vi "SetFrameRate.vi"(8 "error in (no error)":errorcluster, 10 "Frame Rate":u8, 11 "CameraTestingBL in":refnum<class "CameraTesting.lvclass">) -> (0 "error out":errorcluster, 3 "CameraTestingBL out":refnum<class "CameraTesting.lvclass">)   [LabVIEW 2020, in "CameraTesting.lvlib" / "CameraTesting.lvclass"]
doc: "Set the frame rate of the camera"
uses:
  CameraTesting.lvclass
  CameraTesting.lvclass/CameraTesting.ctl
  Camera/ICamera/ICamera/ICamera.lvclass
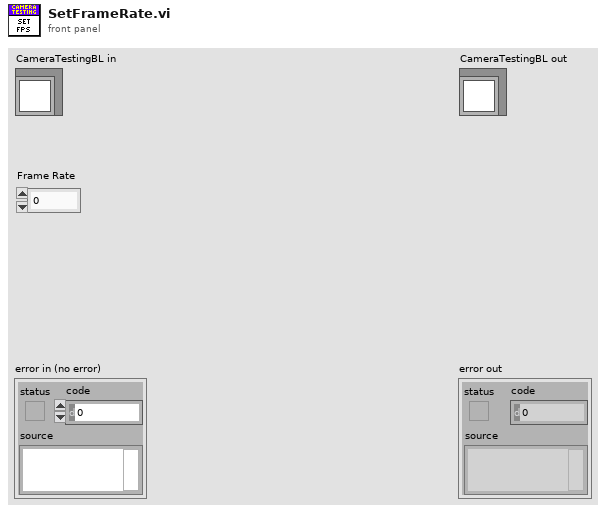
[diagram p1: front panel]
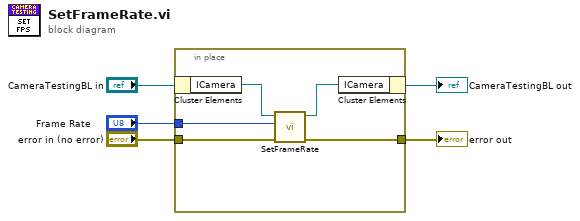
[diagram p0: block diagram]
diagram:
  n1 = in-place {
    in-place-border: "Frame Rate" -> [w10]
    in-place-border: "error in (no error)" -> [w9]
    in-place-border: [w6] -> w2
    n2 = in-place-cluster #1("CameraTestingBL in") -> ("ICamera"=w8:refnum<class "ICamera.lvclass">)
    n3 = call-dynamic "SetFrameRate.vi"("error in (no error)"=w9, "Frame Rate (hex code)"=w10, "ICamera in"=w8) -> ("error out"=w6:errorcluster, "ICamera out"=w7:refnum<class "ICamera.lvclass">)  [unwired: 7 in]
    n4 = in-place-cluster #1("ICamera"=w7) -> (→"CameraTestingBL out":refnum<class "CameraTesting.lvclass">)
  }
  "error out" <- w2
